vi "Washing Machine Program.vi"() -> ()   [LabVIEW 2023]
uses:
  Control 2.ctl
panel:
  in  "On/Off Button":bool
  in  "START":bool
  in  "Mode Of Washing":enum16{"Intensive", "Colourful", "Quick Wash"}(ring)
  out "Time Remaining":dbl
  out "Current Stage":string
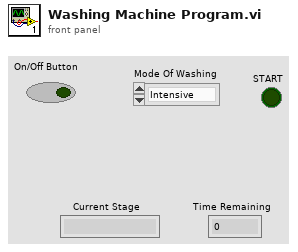
[diagram p1: front panel]
types:
  T1 = typedef "Control 2.ctl" = enum16{"1", "2", "3"}
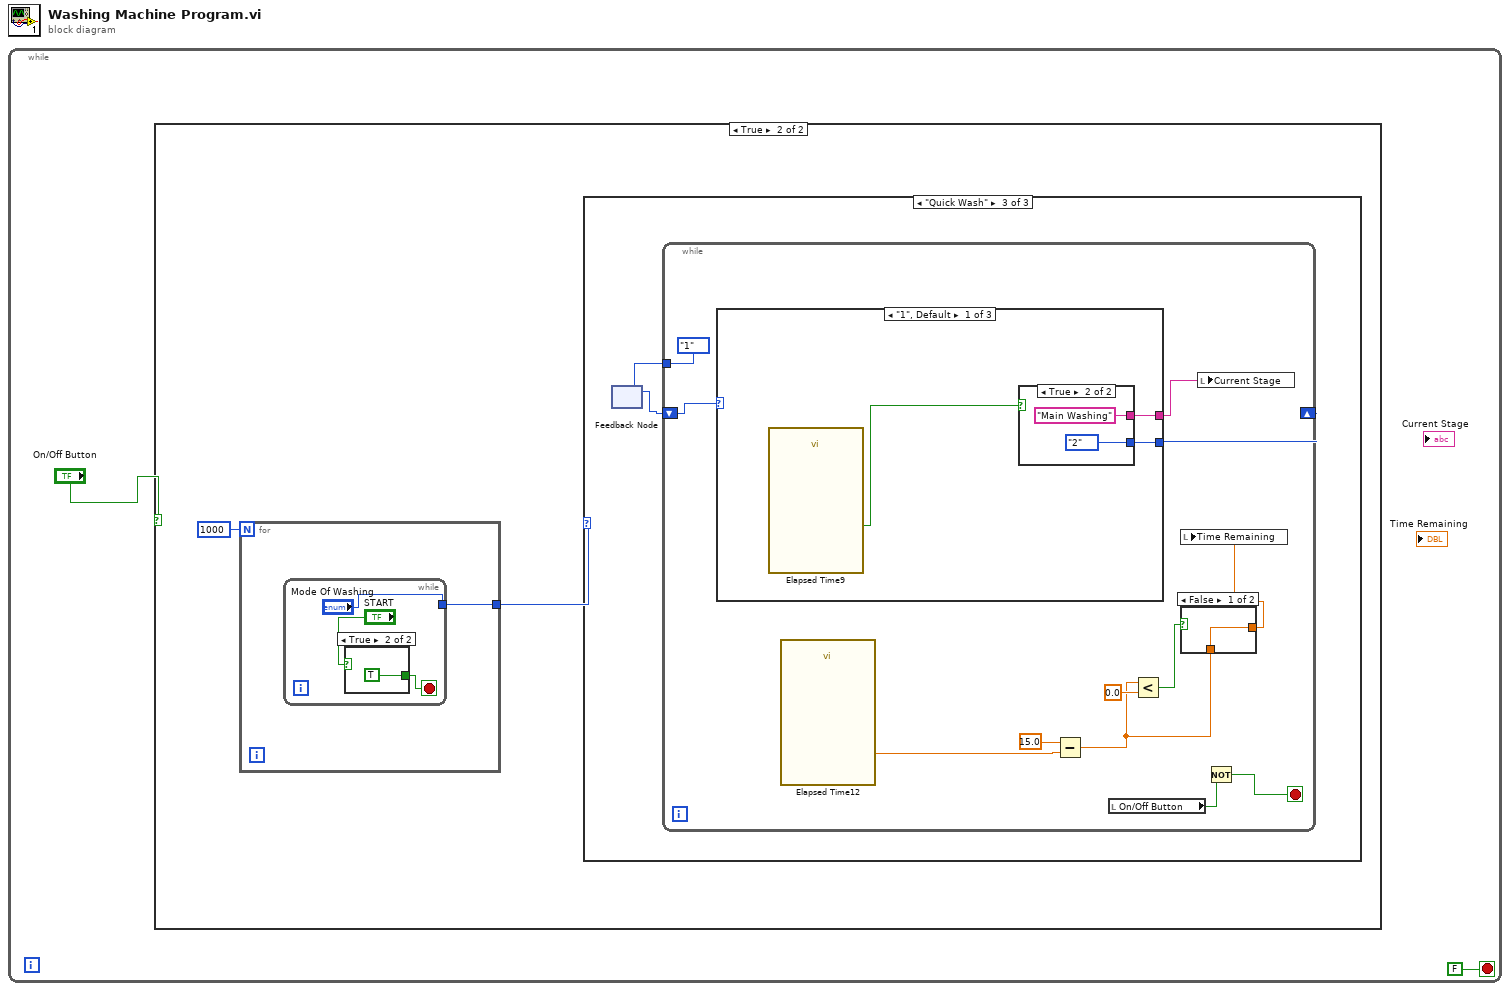
[diagram p0: block diagram]
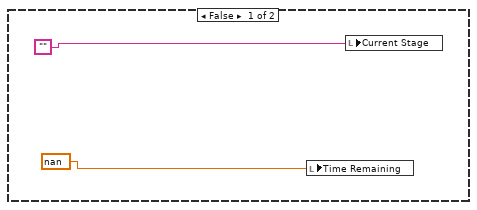
[diagram p2: hidden frame]
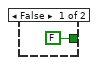
[diagram p3: hidden frame]
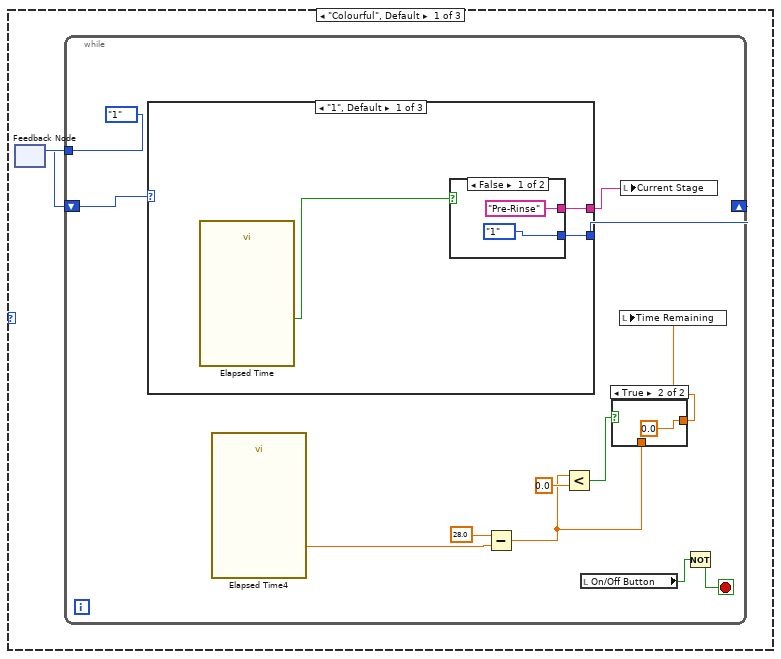
[diagram p4: hidden frame]
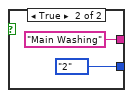
[diagram p6: hidden frame]
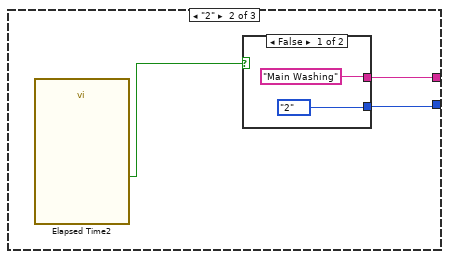
[diagram p7: hidden frame]
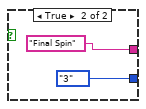
[diagram p8: hidden frame]
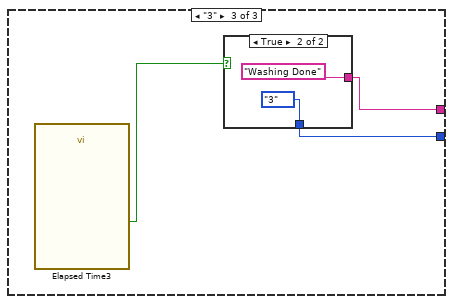
[diagram p9: hidden frame]
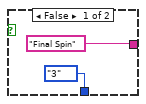
[diagram p10: hidden frame]
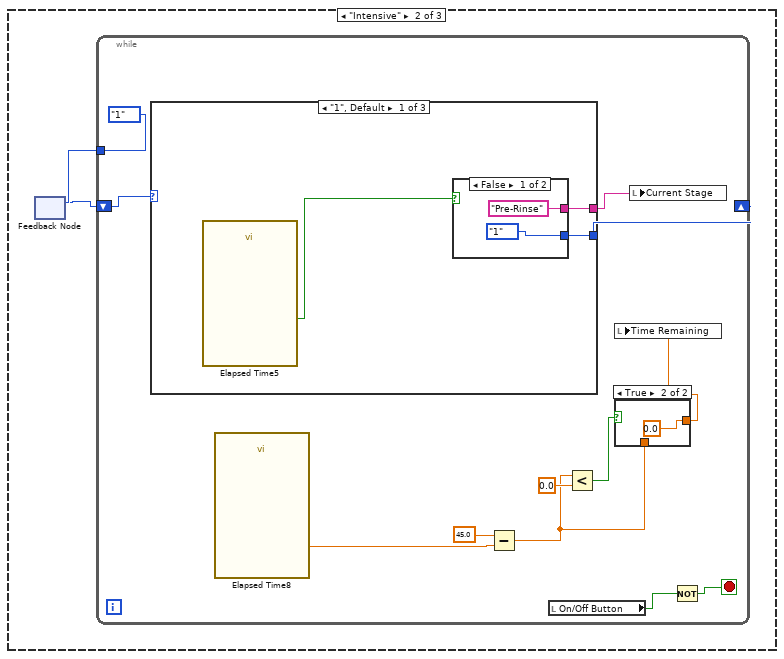
[diagram p11: hidden frame]
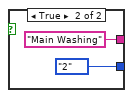
[diagram p13: hidden frame]
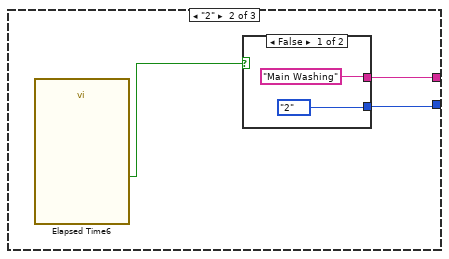
[diagram p14: hidden frame]
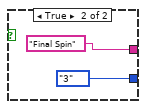
[diagram p15: hidden frame]
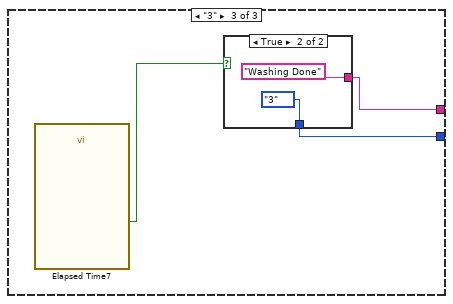
[diagram p16: hidden frame]
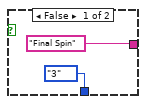
[diagram p17: hidden frame]
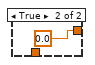
[diagram p18: hidden frame]
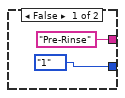
[diagram p19: hidden frame]
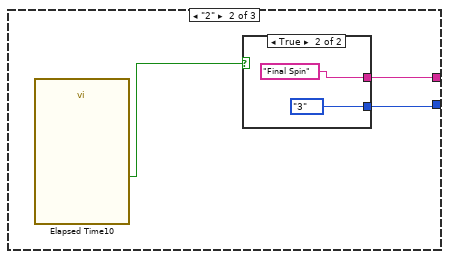
[diagram p20: hidden frame]
diagram:
  n1 = while {
    stop <- FALSE stop-if-true
    n2 = case shown="True" "On/Off Button" {
      frame False {
        n3 = local write "Time Remaining"(nan) -> ()
        n4 = local write "Current Stage"("") -> ()
      }
      frame True {
        n5 = for {
          N: 1000 -> [_]
          tunnel: [w7] -> w5
          n6 = while {
            tunnel: ["Mode Of Washing"] -> w7
            stop <- w10 stop-if-true
            n7 = case shown="True" "START" {
              tunnel: [FALSE TRUE] -> w10
              frame False {
              }
              frame True {
              }
            }
          }
        }
        n8 = case shown="\"Quick Wash\"" w5 {
          frame "Colourful", Default {
            n9 = feedback #1() -> (w13:T1)  [unwired: 1 in]
            n10 = while {
              shift-right: [w22] -> _
              shift-left: w13 -> [w20]
              tunnel: [Control_2."1"] -> w14
              stop <- w16 stop-if-true
              n11 = case shown="\"1\", Default" w20 {
                tunnel: [w31 w37 w45] -> w18
                tunnel: [w30 w36 w43] -> w22
                frame "1", Default {
                  n12 = call "Elapsed Time"() -> ("Time has Elapsed"=w29:bool)  [unwired: 12 in, 7 out]
                  n13 = case shown="False" w29 {
                    tunnel: ["Pre-Rinse" "Main Washing"] -> w31
                    tunnel: [Control_2."1" Control_2."2"] -> w30
                    frame False {
                    }
                    frame True {
                    }
                  }
                }
                frame "2" {
                  n14 = call "Elapsed Time2"() -> ("Time has Elapsed"=w38:bool)  [unwired: 12 in, 7 out]
                  n15 = case shown="False" w38 {
                    tunnel: ["Main Washing" "Final Spin"] -> w37
                    tunnel: [Control_2."2" Control_2."3"] -> w36
                    frame False {
                    }
                    frame True {
                    }
                  }
                }
                frame "3" {
                  n16 = call "Elapsed Time3"() -> ("Time has Elapsed"=w44:bool)  [unwired: 12 in, 7 out]
                  n17 = case shown="True" w44 {
                    tunnel: ["Final Spin" "Washing Done"] -> w45
                    tunnel: [Control_2."3" Control_2."3"] -> w43
                    frame False {
                    }
                    frame True {
                    }
                  }
                }
              }
              n18 = call "Elapsed Time4"() -> ("Elapsed Time (s)"=w26:dbl)  [unwired: 12 in, 7 out]
              n19 = Subtract(x=28.0, y=w26) -> (x-y=w23:dbl)
              n20 = Less?(x=w23, y=0.0) -> (x < y?=w24:bool)
              n21 = local read "On/Off Button"() -> (w15:bool)
              n22 = case shown="True" w24 {
                tunnel: [w27 0.0] -> w17
                tunnel: w23 -> [w27 _]
                frame False {
                }
                frame True {
                }
              }
              n23 = local write "Time Remaining"(w17) -> ()
              n24 = local write "Current Stage"(w18) -> ()
              n25 = Not(x=w15) -> (.not. x?=w16:bool)
            }
            n26 = feedback-in #1(w14) -> ()
          }
          frame "Intensive" {
            n27 = feedback #2() -> (w50:T1)  [unwired: 1 in]
            n28 = while {
              shift-right: [w59] -> _
              shift-left: w50 -> [w57]
              tunnel: [Control_2."1"] -> w51
              stop <- w52 stop-if-true
              n29 = case shown="\"1\", Default" w57 {
                tunnel: [w68 w74 w82] -> w55
                tunnel: [w67 w73 w80] -> w59
                frame "1", Default {
                  n30 = call "Elapsed Time5"() -> ("Time has Elapsed"=w66:bool)  [unwired: 12 in, 7 out]
                  n31 = case shown="False" w66 {
                    tunnel: ["Pre-Rinse" "Main Washing"] -> w68
                    tunnel: [Control_2."1" Control_2."2"] -> w67
                    frame False {
                    }
                    frame True {
                    }
                  }
                }
                frame "2" {
                  n32 = call "Elapsed Time6"() -> ("Time has Elapsed"=w75:bool)  [unwired: 12 in, 7 out]
                  n33 = case shown="False" w75 {
                    tunnel: ["Main Washing" "Final Spin"] -> w74
                    tunnel: [Control_2."2" Control_2."3"] -> w73
                    frame False {
                    }
                    frame True {
                    }
                  }
                }
                frame "3" {
                  n34 = call "Elapsed Time7"() -> ("Time has Elapsed"=w81:bool)  [unwired: 12 in, 7 out]
                  n35 = case shown="True" w81 {
                    tunnel: ["Final Spin" "Washing Done"] -> w82
                    tunnel: [Control_2."3" Control_2."3"] -> w80
                    frame False {
                    }
                    frame True {
                    }
                  }
                }
              }
              n36 = call "Elapsed Time8"() -> ("Elapsed Time (s)"=w63:dbl)  [unwired: 12 in, 7 out]
              n37 = Subtract(x=45.0, y=w63) -> (x-y=w60:dbl)
              n38 = local read "On/Off Button"() -> (w53:bool)
              n39 = Less?(x=w60, y=0.0) -> (x < y?=w61:bool)
              n40 = case shown="True" w61 {
                tunnel: [w64 0.0] -> w54
                tunnel: w60 -> [w64 _]
                frame False {
                }
                frame True {
                }
              }
              n41 = local write "Time Remaining"(w54) -> ()
              n42 = local write "Current Stage"(w55) -> ()
              n43 = Not(x=w53) -> (.not. x?=w52:bool)
            }
            n44 = feedback-in #2(w51) -> ()
          }
          frame "Quick Wash" {
            n45 = feedback #3() -> (w87:T1)  [unwired: 1 in]
            n46 = while {
              shift-right: [w96] -> _
              shift-left: w87 -> [w95]
              tunnel: [Control_2."1"] -> w88
              stop <- w91 stop-if-true
              n47 = case shown="\"1\", Default" w95 {
                tunnel: [w105 w111 w119] -> w93
                tunnel: [w104 w110 w117] -> w96
                frame "1", Default {
                  n48 = call "Elapsed Time9"() -> ("Time has Elapsed"=w103:bool)  [unwired: 12 in, 7 out]
                  n49 = case shown="True" w103 {
                    tunnel: ["Pre-Rinse" "Main Washing"] -> w105
                    tunnel: [Control_2."1" Control_2."2"] -> w104
                    frame False {
                    }
                    frame True {
                    }
                  }
                }
                frame "2" {
                  n50 = call "Elapsed Time10"() -> ("Time has Elapsed"=w112:bool)  [unwired: 12 in, 7 out]
                  n51 = case shown="True" w112 {
                    tunnel: ["Main Washing" "Final Spin"] -> w111
                    tunnel: [Control_2."2" Control_2."3"] -> w110
                    frame False {
                    }
                    frame True {
                    }
                  }
                }
                frame "3" {
                  n52 = call "Elapsed Time11"() -> ("Time has Elapsed"=w118:bool)  [unwired: 12 in, 7 out]
                  n53 = case shown="True" w118 {
                    tunnel: ["Final Spin" "Washing Done"] -> w119
                    tunnel: [Control_2."3" Control_2."3"] -> w117
                    frame False {
                    }
                    frame True {
                    }
                  }
                }
              }
              n54 = call "Elapsed Time12"() -> ("Elapsed Time (s)"=w100:dbl)  [unwired: 12 in, 7 out]
              n55 = Subtract(x=15.0, y=w100) -> (x-y=w97:dbl)
              n56 = local read "On/Off Button"() -> (w90:bool)
              n57 = Less?(x=w97, y=0.0) -> (x < y?=w98:bool)
              n58 = case shown="False" w98 {
                tunnel: [w101 0.0] -> w92
                tunnel: w97 -> [w101 _]
                frame False {
                }
                frame True {
                }
              }
              n59 = local write "Time Remaining"(w92) -> ()
              n60 = local write "Current Stage"(w93) -> ()
              n61 = Not(x=w90) -> (.not. x?=w91:bool)
            }
            n62 = feedback-in #3(w88) -> ()
          }
        }
      }
    }
  }
